vi "variant2Attributes.vi"(0 "HGV_PVBase":refnum<class "HGF_DSCCommand.lvclass">, 2 "rawData":variant, 3 "typeDescriptor":string, 5 "error in (no error)":errorcluster) -> (14 "HGV_PVBase":refnum<class "HGF_DSCCommand.lvclass">, 15 "no link":bool, 16 "Parameter":variant, 17 "typeDescriptor":string, 19 "error out":errorcluster)   [LabVIEW 2012, in "HGF_DSC.lvlib" / "HGF_DSCCommand.lvclass"]
doc: "Convert raw data value of variant to variant attributes Pn, n=0,1,2,..."
uses:
  HGF_DSCCommand.lvclass
  HGF_SV/HGF_SVCommand/HGF_SVCommand.lvclass
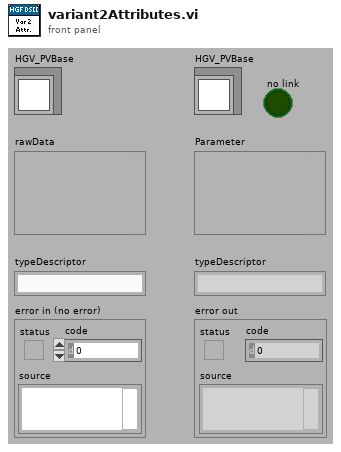
[diagram p1: front panel]
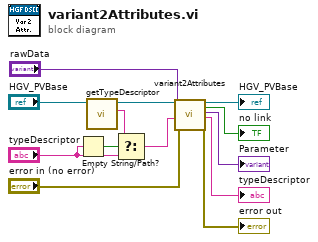
[diagram p0: block diagram]
diagram:
  n1 = Empty String/Path?(string/path="typeDescriptor") -> (empty?=w3:bool)
  n2 = call-dynamic "getTypeDescriptor.vi"("HGF_DSCCommand.lvclass in"="HGV_PVBase") -> ("typeDescriptor"=w1:string, "HGF_DSCCommand.lvclass out"=w6:refnum<class "HGF_DSCCommand.lvclass">)  [unwired: 1 in, 8 out]
  n3 = Select(t=w1, s=w3, f="typeDescriptor") -> (s? t:f=w4:string)
  n4 = call-parent "variant2Attributes.vi"("HGV_PVBase"=w6, "rawData"="rawData", "typeDescriptor"=w4, "error in (no error)"="error in (no error)") -> ("HGV_PVBase"=→"HGV_PVBase":refnum<class "HGF_DSCCommand.lvclass">, "no link"=→"no link":bool, "Parameter"=→"Parameter":variant, "typeDescriptor"=→"typeDescriptor":string, "error out"=→"error out":errorcluster)  [unwired: 11 out]
